vi "CPP-5168PuffReleaseAnalysis.vi"() -> (5 "Plug in titles":string[](array[string]), 7 "Plug in values":string[](array[string]))   [LabVIEW 2012]
uses:
  Controls/Post_Process.ctl
  Globals/Meas_global.vi
  <vilib>/measure/mascope.llb/Transition Measurements 1 chan.vi
  <vilib>/measure/NI_MAPro.lvlib
  <vilib>/Analysis/NI_AALBase.lvlib
panel:
  out "SampleLength":i32
  in  "MedianFilter(points)":i32=3
  in  "PufferCard":tag="PXI1Slot2"
  out "FID2decayConstant":dbl
  out "FID1decayConstant":dbl
  out "FFID1 2":cluster{dbl, dbl, dbl[]}[](graph)
  out "Valve":cluster{dbl, dbl, dbl[]}(graph)
  out "ValveShutAt":dbl format="%.2f"
  out "FFID2":T1(graph)
  out "Current Block No":i32
  out "FFID1":cluster{dbl, dbl, dbl[]}[](graph)
  out "SourceOffIndex":i32
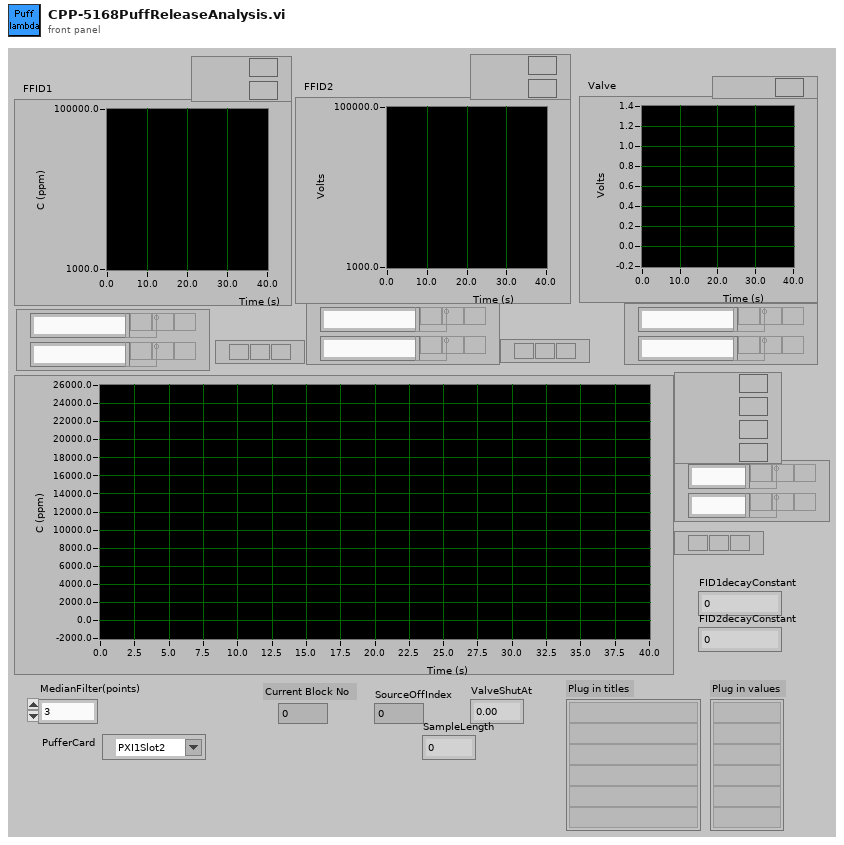
[diagram p1: front panel]
types:
  T1 = cluster{dbl, "SamplingRate":dbl, "Best Exponential Fit":dbl[]}[]
  T2 = cluster{"Weighting":dbl[], "Time (ms)":dbl[], "Voltage":dbl[], "Eng Values":dbl[]}[]
  T3 = typedef "Post_Process.ctl" = enum16{"Take New Data", "Post Process Raw Data File"}
  T4 = cluster{"start time":dbl, "end time":dbl, "ref levels":cluster{"high ref level":dbl, "mid ref level":dbl, "low ref level":dbl, "ref units":u16}}
  T5 = cluster{dbl, "SamplingRate":dbl, "Best Exponential Fit":dbl[]}
  T6 = cluster{dbl, "SamplingRate":dbl, "Filtered X":dbl[]}[]
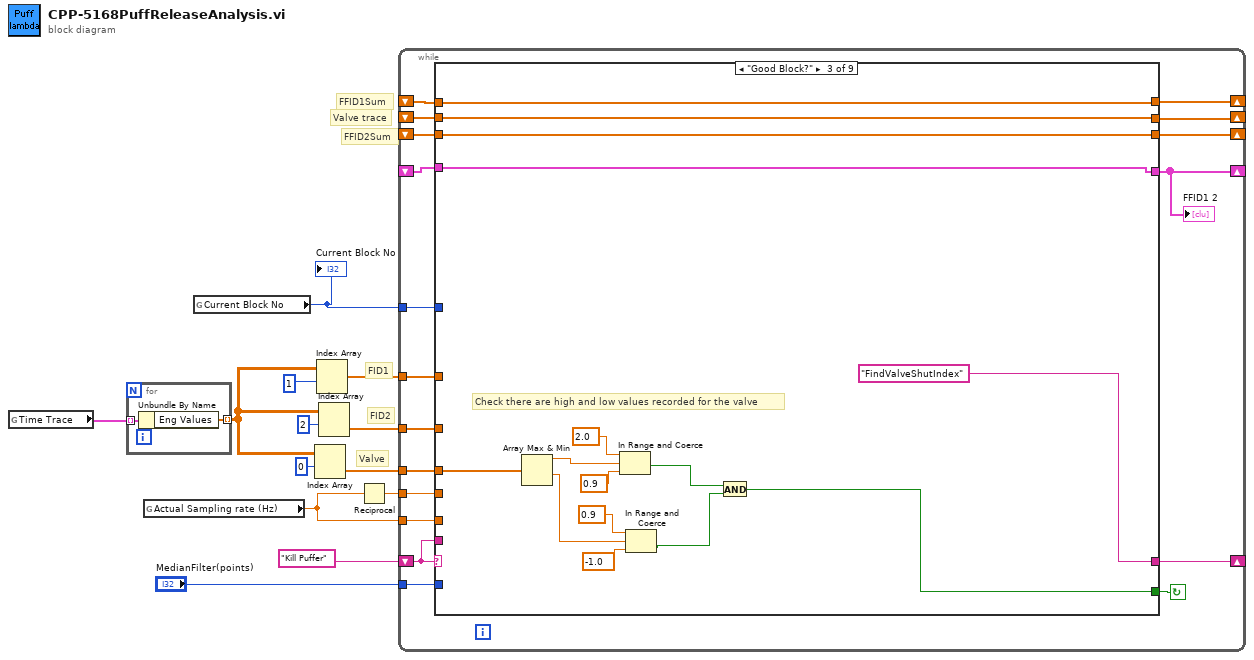
[diagram p0: block diagram]
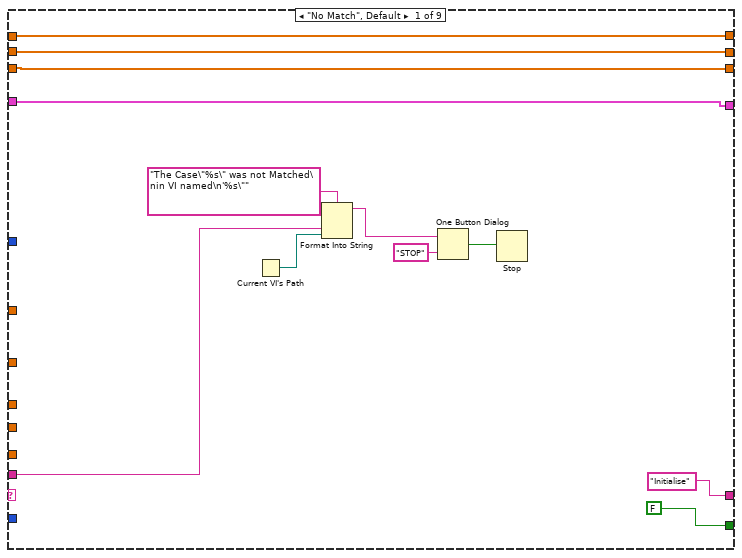
[diagram p2: hidden frame]
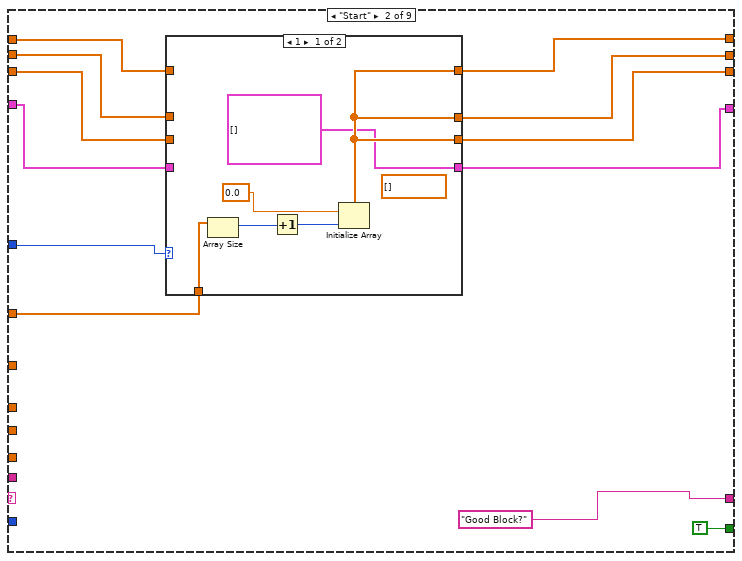
[diagram p3: hidden frame]
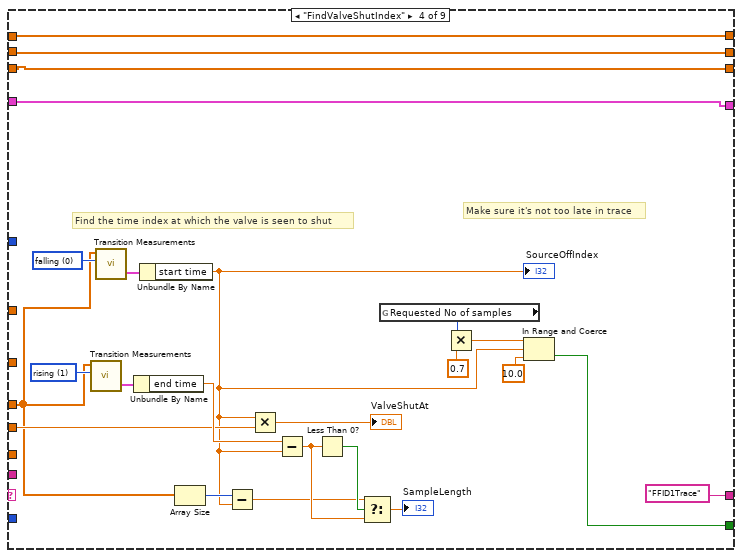
[diagram p5: hidden frame]
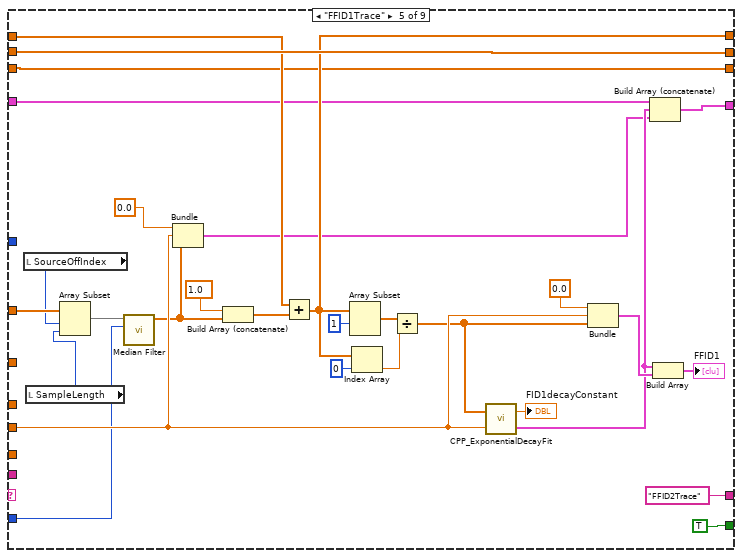
[diagram p6: hidden frame]
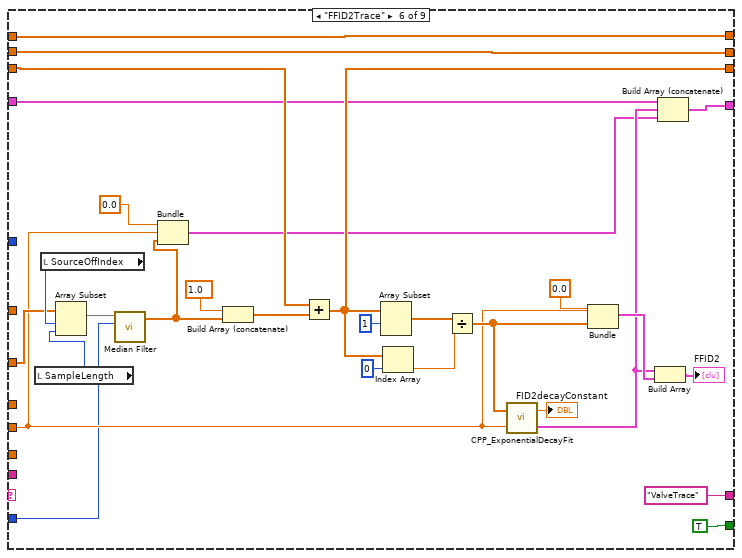
[diagram p7: hidden frame]
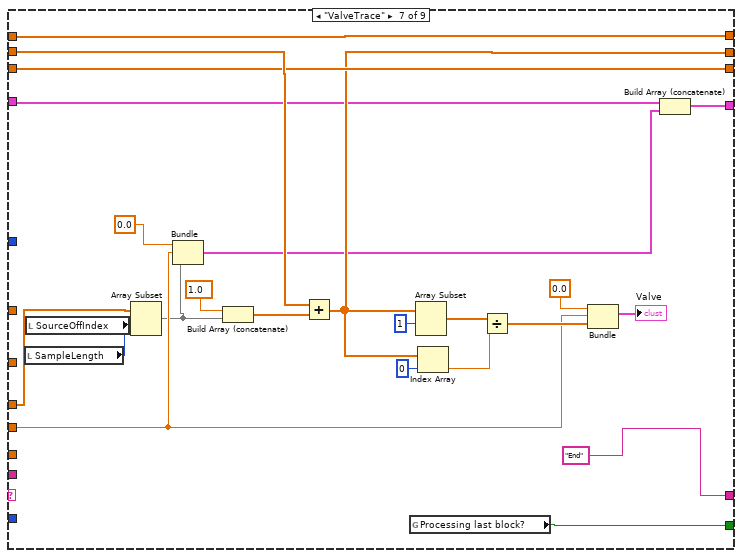
[diagram p8: hidden frame]
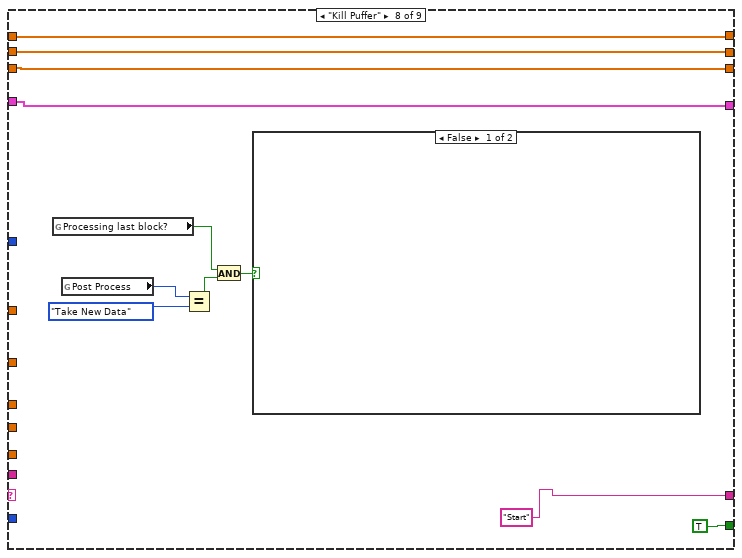
[diagram p9: hidden frame]
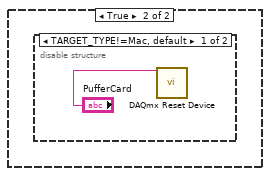
[diagram p10: hidden frame]
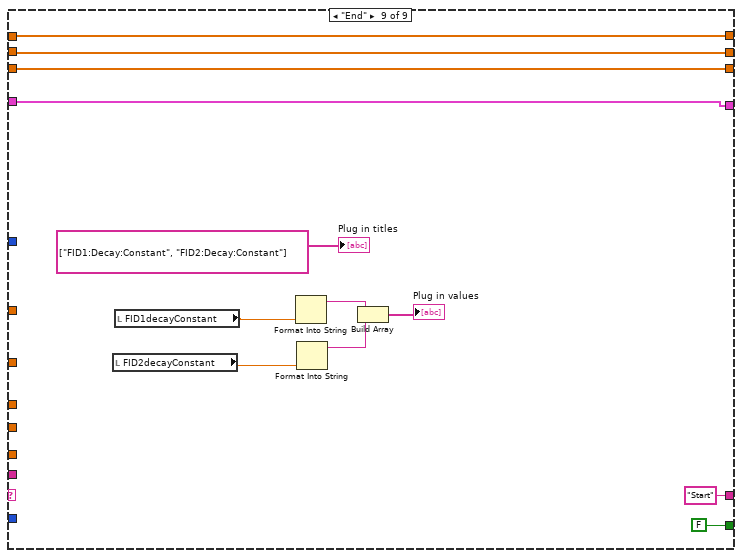
[diagram p12: hidden frame]
diagram:
  # "Valve"
  # "FID2"
  # "FID1"
  # "FFID2Sum"
  # "Valve trace"
  # "FFID1Sum"
  n1 = global read "Meas_global.vi" "Time Trace"() -> (w2:T2)
  n2 = for {
    tunnel: w2 -> [w15] mode=indexing
    tunnel: [w14] -> w1 mode=indexing
    n3 = Unbundle By Name(w15) -> ("Eng Values"=w14:dbl[])
  }
  n4 = global read "Meas_global.vi" "Actual Sampling rate (Hz)"() -> (w5:dbl)
  n5 = global read "Meas_global.vi" "Current Block No"() -> (w10:i32)
  "Current Block No" <- w10
  n6 = Index Array(array=w1, index (row)=0) -> (element=w7:dbl[])  [unwired: 1 in]
  n7 = Index Array(array=w1, index (row)=1) -> (element=w11:dbl[])  [unwired: 1 in]
  n8 = Index Array(array=w1, index (row)=2) -> (element=w12:dbl[])  [unwired: 1 in]
  n9 = Reciprocal(x=w5) -> (1/x=w4:dbl)
  n10 = while {
    shift-left: "Kill Puffer" -> [w31]
    shift-right: [w32] -> _
    shift-right: [w30] -> _
    shift-left: _ -> [w27]
    shift-right: [w29] -> _
    shift-left: _ -> [w28]
    tunnel: w12 -> [w26]
    tunnel: w11 -> [w25]
    tunnel: w5 -> [w24]
    tunnel: w10 -> [w23]
    shift-right: [w21] -> _
    shift-left: _ -> [w20]
    tunnel: w7 -> [w22]
    tunnel: w4 -> [w19]
    shift-right: [w17] -> _
    shift-left: _ -> [w18]
    tunnel: "MedianFilter(points)" -> [w16]
    stop <- w33 continue-if-true
    n11 = case shown="\"Good Block?\"" w31 {
      tunnel: [FALSE TRUE ("Processing last block?") w77 w97 TRUE ("Processing last block?") TRUE ("Processing last block?") w167 TRUE ("Processing last block?") FALSE ("Processing last block?")] -> w33
      tunnel: ["Initialise" "Good Block?" "FindValveShutIndex" "FFID1Trace" "FFID2Trace" "ValveTrace" "End" "Start" "Start" ("f")] -> w32
      tunnel: w31 -> [w40 _ _ _ _ _ _ _ _]
      tunnel: [w37 w56 w82 w105 w125 w152 w179 w199 w212] -> w30
      tunnel: [w36 w54 w81 w104 w133 w162 w176 w198 w211] -> w29
      tunnel: w28 -> [w36 w53 w81 w104 w133 w162 w178 w198 w211]
      tunnel: w27 -> [w37 w55 w82 w105 w131 w152 w179 w199 w212]
      tunnel: w26 -> [_ _ _ _ _ w153 _ _ _]
      tunnel: w25 -> [_ w52 _ _ w132 _ _ _ _]
      tunnel: w24 -> [_ _ _ _ _ _ _ _ _]
      tunnel: w23 -> [_ w51 _ _ _ _ _ _ _]
      tunnel: w22 -> [_ _ w73 w86 _ _ w175 _ _]
      tunnel: [w35 w50 w74 w103 w122 w150 w177 w194 w210] -> w21
      tunnel: w20 -> [w35 w49 w74 w103 w122 w151 w177 w194 w210]
      tunnel: w19 -> [_ _ _ w90 w116 w143 w170 _ _]
      tunnel: [w34 w47 w68 w95 w120 w149 w174 w190 w207] -> w17
      tunnel: w18 -> [w34 w46 w68 w95 w121 w148 w173 w190 w207]
      tunnel: w16 -> [_ _ _ _ w108 w137 _ _ _]
      frame "No Match", Default {
        n12 = Current VI's Path() -> (path=w39:path)
        n13 = Format Into String(format string="The Case\"%s\" was not Matched\nin VI named\n'%s\"" ("Format String"), w40, w39) -> (resulting string=w43:string)  [unwired: 2 in, 1 out]
        n14 = One Button Dialog(message=w43, button name ("OK")="STOP") -> (true=w41:bool)
        n15 = Stop(stop? (T)=w41) -> ()
      }
      frame "Start" {
        n16 = case shown="1" w51 {
          tunnel: [w60 w67] -> w56
          tunnel: w55 -> [_ w67]
          tunnel: [w60 w66] -> w54
          tunnel: w53 -> [_ w66]
          tunnel: w52 -> [w63 _]
          tunnel: [w60 w65] -> w50
          tunnel: w49 -> [_ w65]
          tunnel: [cluster{dbl, dbl, dbl[]}[] [] w64] -> w47
          tunnel: w46 -> [_ w64]
          frame 1 {
            (unwired) dbl[] []
            n17 = Array Size(array=w63) -> (size(s)=w62:i32)
            n18 = Increment(x=w62) -> (x+1=w59:i32)
            n19 = Initialize Array(0.0 ("element"), w59) -> (w60:dbl[])
          }
          frame 2, Default {
          }
        }
      }
      frame "Good Block?" {
        # "Check there are high and low values recorded for the valve"
        n20 = Array Max & Min(array=w73) -> (max value=w76:dbl, min value=w70:dbl)  [unwired: 2 out]
        n21 = In Range and Coerce(upper limit=2.0, x=w76, lower limit=0.9 ("y")) -> (In Range?=w78:bool)  [unwired: 1 out]
        n22 = In Range and Coerce(upper limit=0.9, x=w70, lower limit=-1.0 ("y")) -> (In Range?=w69:bool)  [unwired: 1 out]
        n23 = And(x=w78, y=w69) -> (x .and. y?=w77:bool)
      }
      frame "FindValveShutIndex" {
        w92 = u16 0 items=["falling", "rising"] ("polarity (rising)")
        w93 = u16 1 items=["falling", "rising"] ("polarity (rising)")
        # "Make sure it's not too late in trace"
        # "Find the time index at which the valve is seen to shut"
        n24 = call-poly <vilib>:"Transition Measurements.vi"("polarity (rising)"=w93, "signal in"=w86) -> ("measurement info"=w94:T4)  [unwired: 4 in, 5 out]
        n25 = call-poly <vilib>:"Transition Measurements.vi"("polarity (rising)"=w92, "signal in"=w86) -> ("measurement info"=w102:T4)  [unwired: 4 in, 5 out]
        n26 = Unbundle By Name(w94) -> ("end time"=w91:dbl)
        n27 = Unbundle By Name(w102) -> ("start time"=w84:dbl)
        "SourceOffIndex" <- w84
        n28 = Array Size(array=w86) -> (size(s)=w85:i32)
        n29 = Subtract(x=w85, y=w84) -> (x-y=w83:dbl)
        n30 = Multiply(x=w84, y=w90) -> (x*y=→"ValveShutAt":dbl)
        n31 = Subtract(x=w91, y=w84) -> (x-y=w88:dbl)
        n32 = Less Than 0?(x=w88) -> (x < 0?=w89:bool)
        n33 = Select(t=w83, s=w89, f=w88) -> (s? t:f=→"SampleLength":dbl)
        n34 = global read "Meas_global.vi" "Requested No of samples"() -> (w101:i32)
        n35 = Multiply(x=w101, y=0.7 ("lower limit")) -> (x*y=w99:dbl)
        n36 = In Range and Coerce(upper limit=w99, x=w84, lower limit=10.0) -> (In Range?=w97:bool)  [unwired: 1 out]
      }
      frame "FFID1Trace" {
        n37 = local read "SourceOffIndex"() -> (w128:i32)
        n38 = local read "SampleLength"() -> (w107:i32)
        n39 = Array Subset(array=w132, index=w128, length=w107) -> (w109:dbl[])
        n40 = call <vilib>:"Median Filter.vi"("left rank"=w108, "X"=w109) -> ("Filtered X"=w110:dbl[])  [unwired: 8 in, 1 out]
        n41 = Bundle(0.0, w116, "Filtered X"=w110) -> (w112:cluster{dbl, dbl, "Filtered X":dbl[]})  [unwired: 1 out]
        n42 = Build Array (concatenate)(1.0, w110) -> (w129:dbl[])
        n43 = Add(x=w131, y=w129) -> (x+y=w125:dbl[])
        n44 = Array Subset(array=w125, index=1) -> (w124:dbl[])  [unwired: 1 in]
        n45 = Index Array(array=w125, index=0) -> (element=w123:dbl)
        n46 = Divide(x=w124, y=w123) -> (x/y=w111:dbl[])
        n47 = call "CPP_ExponentialDecayFit.vi"("SamplingRate"=w116, "DecayData"=w111) -> ("graphCluster"=w113:T5, "decayConstant"=→"FID1decayConstant":dbl)
        n48 = Bundle(0.0, w116, w111) -> (w114:cluster{dbl, dbl, dbl[]})  [unwired: 1 out]
        n49 = Build Array (concatenate)(w121, w113, w112) -> (w120:T6)
        n50 = Build Array(w113, w114) -> (→"FFID1":T1)
      }
      frame "FFID2Trace" {
        n51 = local read "SampleLength"() -> (w136:i32)
        n52 = local read "SourceOffIndex"() -> (w159:i32)
        n53 = Array Subset(array=w153, index=w159, length=w136) -> (w138:dbl[])
        n54 = call <vilib>:"Median Filter.vi"("left rank"=w137, "X"=w138) -> ("Filtered X"=w139:dbl[])  [unwired: 8 in, 1 out]
        n55 = Bundle(0.0, w143, "Filtered X"=w139) -> (w140:cluster{dbl, dbl, "Filtered X":dbl[]})  [unwired: 1 out]
        n56 = Build Array (concatenate)(1.0, w139) -> (w160:dbl[])
        n57 = Add(x=w151, y=w160) -> (x+y=w150:dbl[])
        n58 = Array Subset(array=w150, index=1) -> (w155:dbl[])  [unwired: 1 in]
        n59 = Index Array(array=w150, index=0) -> (element=w154:dbl)
        n60 = Divide(x=w155, y=w154) -> (x/y=w144:dbl[])
        n61 = call "CPP_ExponentialDecayFit.vi"("SamplingRate"=w143, "DecayData"=w144) -> ("graphCluster"=w141:T5, "decayConstant"=→"FID2decayConstant":dbl)
        n62 = Bundle(0.0, w143, w144) -> (w142:cluster{dbl, dbl, dbl[]})  [unwired: 1 out]
        n63 = Build Array(w141, w142) -> (→"FFID2":T1)
        n64 = Build Array (concatenate)(w148, w141, w140) -> (w149:T6)
      }
      frame "ValveTrace" {
        n65 = local read "SampleLength"() -> (w165:i32)
        n66 = local read "SourceOffIndex"() -> (w186:i32)
        n67 = Array Subset(array=w175, index=w186, length=w165) -> (w169:dbl[])
        n68 = Bundle(0.0, w170, w169) -> (w168:cluster{dbl, dbl, dbl[]})  [unwired: 1 out]
        n69 = Build Array (concatenate)(1.0, w169) -> (w187:dbl[])
        n70 = Add(x=w178, y=w187) -> (x+y=w176:dbl[])
        n71 = global read "Meas_global.vi" "Processing last block?"() -> (w167:bool)
        n72 = Array Subset(array=w176, index=1) -> (w181:dbl[])  [unwired: 1 in]
        n73 = Index Array(array=w176, index=0) -> (element=w180:dbl)
        n74 = Divide(x=w181, y=w180) -> (x/y=w185:dbl[])
        n75 = Bundle(0.0, w170, w185) -> (→"Valve":cluster{dbl, dbl, dbl[]})  [unwired: 1 out]
        n76 = Build Array (concatenate)(w173, w168) -> (w174:T6)
      }
      frame "Kill Puffer" {
        n77 = global read "Meas_global.vi" "Processing last block?"() -> (w193:bool)
        n78 = global read "Meas_global.vi" "Post Process"() -> (w196:T3)
        n79 = Equal?(x=w196, y=Post_Process."Take New Data" ("Post Process")) -> (x = y?=w192:bool)
        n80 = And(x=w193, y=w192) -> (x .and. y?=w191:bool)
        n81 = case shown="False" w191 {
          frame False {
          }
          frame True {
            n82 = disable-structure shown="TARGET_TYPE!=Mac, default" {
              frame condition #0 (active) {
                n83 = call <vilib>:"DAQmx Reset Device.vi"("device in"="PufferCard") -> ()  [unwired: 14 in, 1 out]
              }
              frame condition #1 {
              }
            }
          }
        }
      }
      frame "End" {
        n84 = local read "FID2decayConstant"() -> (w203:dbl)
        n85 = local read "FID1decayConstant"() -> (w205:dbl)
        n86 = Format Into String(w205) -> (resulting string=w204:string)  [unwired: 3 in, 1 out]
        n87 = Format Into String(w203) -> (resulting string=w202:string)  [unwired: 3 in, 1 out]
        n88 = Build Array(w204, w202) -> (→"Plug in values":string[])
        "Plug in titles" <- string[] ["FID1:Decay:Constant", "FID2:Decay:Constant"] ("Plug in titles")
      }
    }
    "FFID1 2" <- w17
  }
